vi "Write Register (Core).vi"(0 "SLSC Remote in":refnum<class "SLSC Remote.lvclass">, 1 "type":enum16{"U8", "U16", "U32", "U64"}(ring), 5 "device":refnum<k21>="$DefaultDevices", 7 "register address":u32 format="%.0x", 9 "data":u64 format="%.0x", 11 "error in (no error)":errorcluster) -> (4 "SLSC Remote out":refnum<class "SLSC Remote.lvclass">, 6 "device out":refnum<k21>, 8 "next register address":u32 format="%.0x", 15 "error out":errorcluster)   [LabVIEW 2016, in "SLSC Interfaces.lvlib" / "SLSC Remote.lvclass"]
uses:
  SLSC Remote.lvclass
  C:/Users/tblair/Documents/Git Projects/SLSC-Interface/Source/SLSC Interface Class/SLSC Interface.lvclass
  <vilib>/National Instruments/JSON Support for LabVIEW/JSON Data Classes/JSON Object/JSON Object.lvclass
  C:/Program Files (x86)/National Instruments/LabVIEW 2016/vi.lib/National Instruments/JSON Support for LabVIEW/JSON Data Classes/JSON Datatype/JSON Datatype.lvclass
  <vilib>/National Instruments/JSON Support for LabVIEW/JSON Data Classes/JSON Object/New JSON Object (Empty).vi
  <vilib>/National Instruments/JSON Support for LabVIEW/JSON Data Classes/JSON Object/Insert Key Value Pair (Single String).vi
  <vilib>/National Instruments/JSON Support for LabVIEW/JSON Data Classes/JSON Object/Insert Key Value Pair (Single Numeric).vi
  <vilib>/NI/NI JSONRPC Server Framework/Classes/Server/Format Client Request (Auto-Increment).vi
  <vilib>/httpClient/POSTBuffer.vi
  <vilib>/National Instruments/JSON Support for LabVIEW/JSON Data Classes/JSON Datatype/To More Specific Type (Object).vi
  <vilib>/National Instruments/JSON Support for LabVIEW/JSON Data Classes/JSON Object/Get Value (Numeric Value).vi
  <vilib>/NI/NI JSONRPC Server Framework/Classes/Server/JSONRPC Server.lvclass
  <vilib>/httpClient/LabVIEWHTTPClient.lvlib
  <vilib>/National Instruments/JSON Support for LabVIEW/JSON Data Classes/JSON Datatype/JSON Datatype.lvclass
  C:/Program Files (x86)/National Instruments/LabVIEW 2016/vi.lib/National Instruments/JSON Support for LabVIEW/JSON Data Classes/JSON Structured Type/JSON Structured Type.lvclass
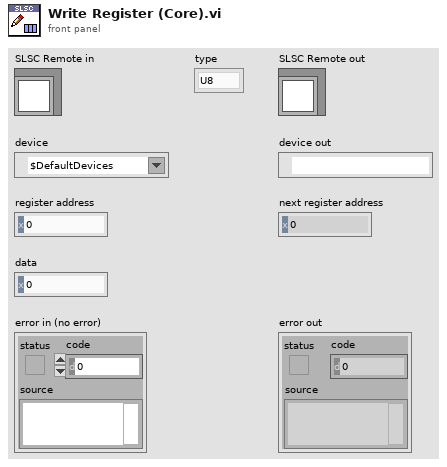
[diagram p1: front panel]
types:
  T1 = typedef "LabVIEWHTTPClient.lvlib/ClientHandle.ctl" = refnum<k1>
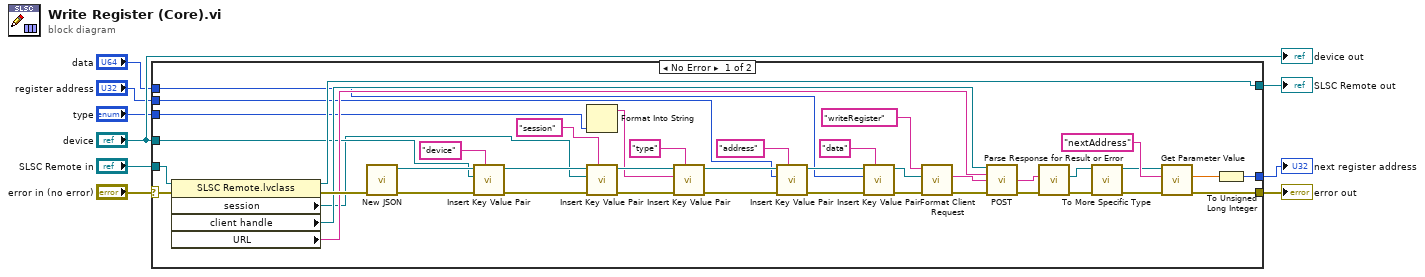
[diagram p0: block diagram]
diagram:
  n1 = case shown="No Error" "error in (no error)" {
    selector: "error in (no error)" -> [w49 w52]
    tunnel: "device" -> [w14 _]
    tunnel: "SLSC Remote in" -> [w51 w53]
    tunnel: [w50 w53] -> w8
    tunnel: [w28 w52] -> w2
    tunnel: "type" -> [w33 _]
    tunnel: "register address" -> [w12 _]
    tunnel: "data" -> [w13 _]
    tunnel: [w27 _] -> w3
    frame No Error {
      n2 = property class="SLSC Remote.lvclass"(reference=w51, error in=w49) -> (reference out=w50:refnum<class "SLSC Remote.lvclass">, error out=w48:errorcluster, "session"=w10:refnum<k21>, "client handle"=w43:T1, "URL"=w42:string)
      n3 = call-poly <vilib>:"New JSON.vi"("error in (no error)"=w48) -> ("error out"=w47:errorcluster, "JSON Object out"=w19:refnum<class "JSON Object.lvclass">)  [unwired: 9 in]
      n4 = call-poly <vilib>:"Insert Key Value Pair.vi"("key"="device" ("Name"), "error in (no error)"=w47, "value"=w14, "JSON Object in"=w19) -> ("error out"=w46:errorcluster, "JSON Object out"=w18:refnum<class "JSON Object.lvclass">)  [unwired: 5 in, 1 out]
      n5 = Format Into String(w33) -> (resulting string=w11:string)  [unwired: 3 in, 1 out]
      n6 = call-poly <vilib>:"Insert Key Value Pair.vi"("key"="session" ("Name"), "error in (no error)"=w46, "value"=w10, "JSON Object in"=w18) -> ("error out"=w34:errorcluster, "JSON Object out"=w17:refnum<class "JSON Object.lvclass">)  [unwired: 5 in, 1 out]
      n7 = call-poly <vilib>:"Insert Key Value Pair.vi"("key"="type" ("Name"), "error in (no error)"=w34, "value"=w11, "JSON Object in"=w17) -> ("error out"=w38:errorcluster, "JSON Object out"=w16:refnum<class "JSON Object.lvclass">)  [unwired: 5 in, 1 out]
      n8 = call-poly <vilib>:"Insert Key Value Pair.vi"("key"="address" ("Name"), "error in (no error)"=w38, "value"=w12, "JSON Object in"=w16) -> ("error out"=w35:errorcluster, "JSON Object out"=w15:refnum<class "JSON Object.lvclass">)  [unwired: 5 in, 1 out]
      n9 = call-poly <vilib>:"Insert Key Value Pair.vi"("key"="data" ("Name"), "error in (no error)"=w35, "value"=w13, "JSON Object in"=w15) -> ("error out"=w37:errorcluster, "JSON Object out"=w36:refnum<class "JSON Object.lvclass">)  [unwired: 5 in, 1 out]
      n10 = call-poly <vilib>:"Format Client Request.vi"("error in (no error)"=w37, "JSON in"=w36, "method"="writeRegister") -> ("error out"=w41:errorcluster, "Request String"=w44:string)  [unwired: 7 in]
      n11 = call-poly <vilib>:"POST.vi"("client handle"=w43, "url"=w42, "buffer"=w44, "error in (no error)"=w41) -> ("body"=w40:string, "error out"=w39:errorcluster)  [unwired: 8 in, 2 out]
      n12 = call <vilib>:"Parse Response for Result or Error.vi"("error in"=w39, "Response String In"=w40) -> ("error out"=w30:errorcluster, "JSON out"=w25:refnum<class "JSON Datatype.lvclass">)  [unwired: 7 in, 1 out]
      n13 = call-poly <vilib>:"To More Specific Type.vi"("error in (no error)"=w30, "JSON Datatype in"=w25) -> ("error out"=w26:errorcluster, "JSON Datatype out"=w24:refnum<class "JSON Object.lvclass">)  [unwired: 8 in]
      n14 = call-poly <vilib>:"Get Parameter Value.vi"("error in (no error)"=w26, "key"="nextAddress" ("Parameter Name"), "JSON Object in"=w24) -> ("error out"=w28:errorcluster, "value"=w23:dbl)  [unwired: 6 in, 1 out]
      n15 = To Unsigned Long Integer(number=w23) -> (unsigned 32bit integer=w27:u32)
    }
    frame Error {
    }
  }
  "error out" <- w2
  "SLSC Remote out" <- w8
  "next register address" <- w3
  "device out" <- "device"
